vi "G#MethodTemplates_SetModifiedAttributes.vi"(0 "reference in":refnum<class "G#MethodTemplates.lvclass">, 2 "attributes":T1, 3 "Only unlock data? (F)":bool, 4 "Unlock data if error? (T)":bool=TRUE, 5 "error in (no error)":errorcluster, 7 "Update data even if error? (F)":bool) -> (14 "reference out":refnum<class "G#MethodTemplates.lvclass">, 19 "error out":errorcluster)   [LabVIEW 2017, in "G#MethodTemplates.lvclass"]
doc: "This VI overwrites the class attributes associated with this class or subclass object reference and unlocks it for write access. If error in is set, the object is unlocked but its data will not be modified. If reference is wired, the class attributes of the class (or sub class) will be affected else the class attributes will default to the class.\n\nIn order to use this VI, you must first successfully lock the object's data using this class GetClassAttributesToModify VI."
uses:
  <vilib>/addons/_AddQ/G#Templates/G#MethodTemplates/G#MethodTemplates.lvclass
  <vilib>/addons/_AddQ/G#Templates/G#MethodTemplates/protected/ObjectAttributes.ctl
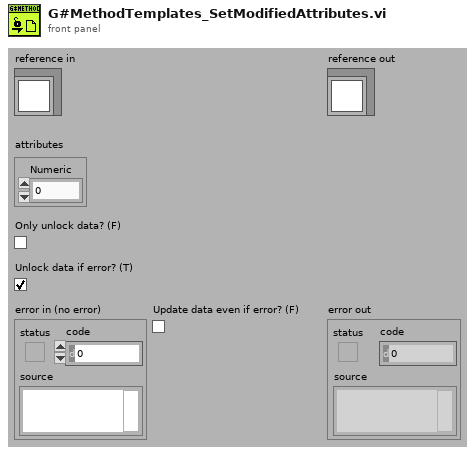
[diagram p1: front panel]
types:
  T1 = typedef "G#MethodTemplates.lvclass/ObjectAttributes.ctl" = cluster{"Numeric":dbl}
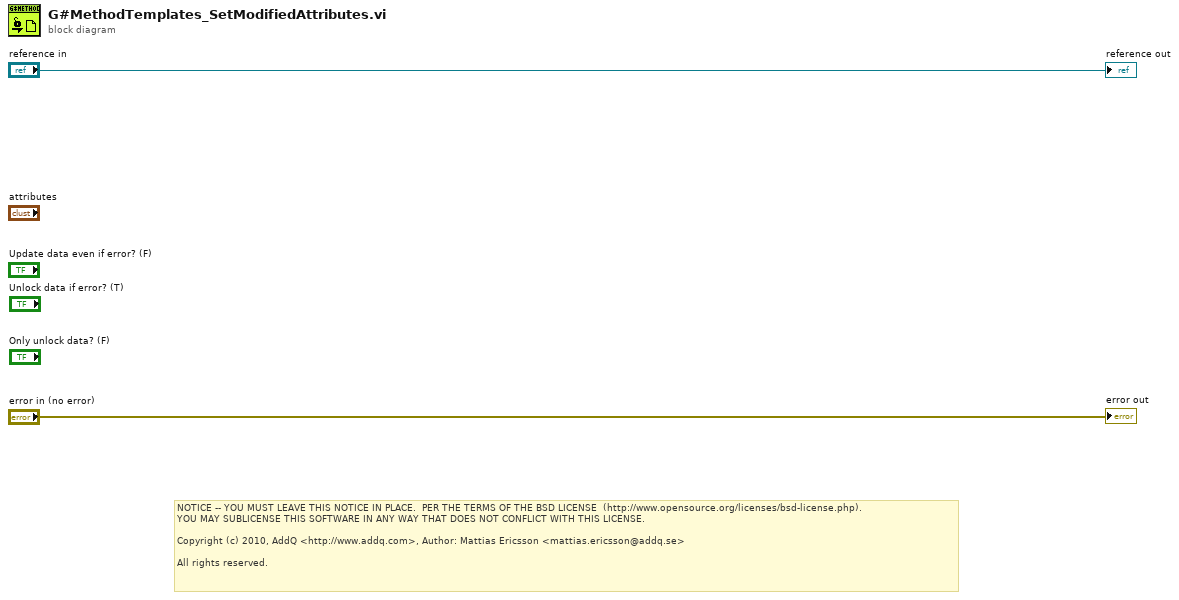
[diagram p0: block diagram]
diagram:
  # "NOTICE -- YOU MUST LEAVE THIS NOTICE IN PLACE.  PER THE TERMS OF THE BSD LICENSE  (http://www.opensource.org/licenses/bsd-license.php).\nYOU MAY SUBLICENSE THIS SOFTWARE IN ANY WAY THAT DOES NOT CONFLICT WITH THIS LICENSE.\n\nCopyright (c) 2010, AddQ <http://www.addq.com>, Author: Mattias Ericsson <mattias.ericsson@addq.se>\n\nAll rights reserved."
  "error out" <- "error in (no error)"
  "reference out" <- "reference in"
